vi "testSegmentation.vi"() -> ()   [LabVIEW 2012]
panel:
  out "Volume":dbl[][][](array[numeric])
  out "ROIs":T1(array[cluster])
  in  "Number of cells":u32=200
  in  "Threshold":u32
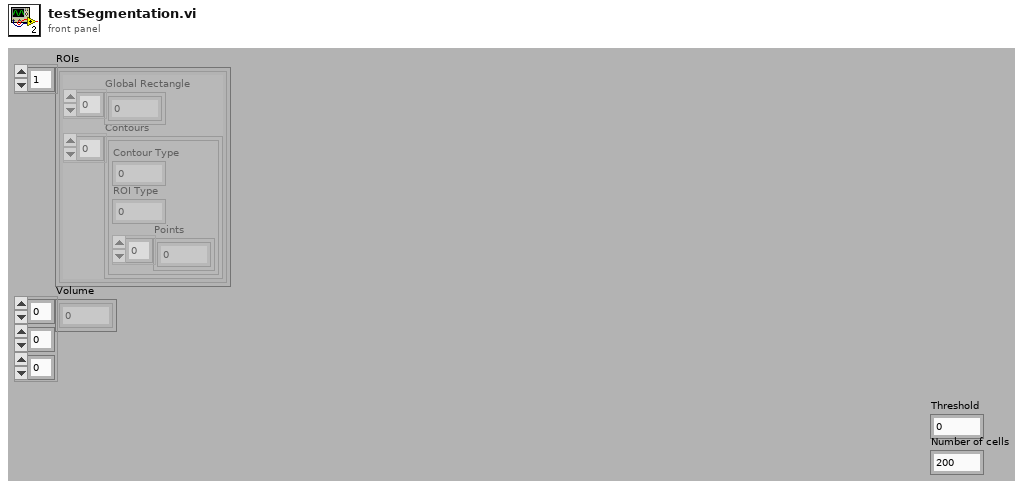
[diagram p1: front panel]
types:
  T1 = cluster{"Global Rectangle":i32[], "Contours":cluster{"Contour Type":u32, "ROI Type":u32, "Points":i32[]}[]}[]
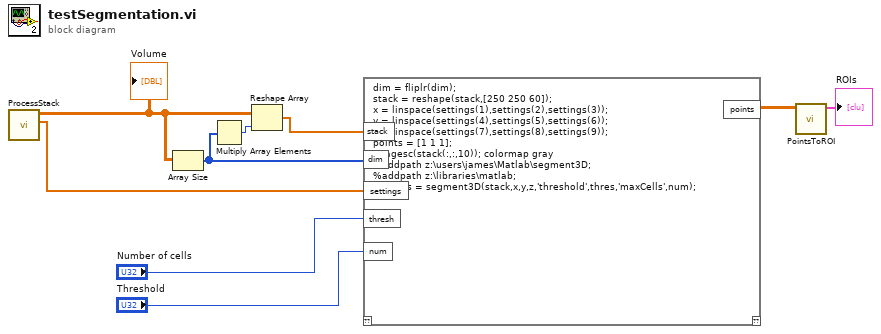
[diagram p0: block diagram]
diagram:
  n1 = call "ProcessStack.vi"() -> ("ScanSettings"=w1:dbl[], "Volume"=w2:dbl[][][])  [unwired: 10 in]
  "Volume" <- w2
  n2 = Array Size(array=w2) -> (size(s)=w9:i32[])
  n3 = Multiply Array Elements(1:w9) -> (0:w8:i32)
  n4 = Reshape Array(w2, w8) -> (w7:dbl[])
  n5 = script code="dim = fliplr(dim);\nstack = reshape(stack,[250 250 60]);\nx = linspace(settings(1),settings(2),settings(3));\ny = linspace(settings(4),settings(5),settings(6));\nz = linspace(settings(7),settings(8),settings(9));\npoints = [1 1 1];\nimagesc(stack(:,:,10)); colormap gray\n%addpath z:\\users\\james\\Matlab\\segment3D;\n%addpath z:\\libraries\\matlab;\n%points = segment3D(stack,x,y,z,'threshold',thres,'maxCells',num);"("stack"=w7, "dim"=w9, "settings"=w1, "thresh"="Number of cells", "num"="Threshold") -> ("points"=w4:cdb[][])  [unwired: 1 in, 1 out]
  n6 = call "PointsToROI.vi"("Points"=w4) -> ("ROIs"=→"ROIs":T1)  [unwired: 10 in]
